vi "Dashboard Main.vi"() -> ()   [LabVIEW 2015]
uses:
  <vilib>/Utility/miscctls.llb/LVRowAndColumnTypeDef.ctl
  <vilib>/event_ctls.llb/eventvkey.ctl
  <vilib>/Rock Robotics/WPI/Dashboard/WPI_DashboardLogging Global.vi
  <vilib>/Rock Robotics/Network Tables/NT Write String Array.vi
  <vilib>/Rock Robotics/Network Tables/NT Read Numeric Array.vi
  <vilib>/Utility/config.llb/Write Key (String).vi
  <vilib>/Utility/config.llb/Write Key (I32).vi
  <vilib>/Rock Robotics/Network Tables/NT Write Boolean.vi
  <vilib>/Rock Robotics/Network Tables/NT Read Boolean.vi
  <vilib>/Utility/config.llb/NI_LVConfig.lvlib
panel:
  in  "TCP":refnum<k5>
  in  "Rec Mode":enum32{"Stop", "Record", "Playback"}(radio)
  in  "Vision":u16(ring) items=["Camera Off", "USB Camera SW", "USB Camera HW", "IP Camera"]
  out "Camera IP":string
  out "Image Message":string="Timeout in Camera Communications"
  in  "Dashboard Tab":T1(tab)
  in  "Select Auto":string(combo)
  out "NT Connection":bool
  in  "Camera Settings":T2={"Frame Rate"=30, "Compression"=30, "Size"=1} {"Frame Rate" scale=1.0..30.0; "Size" items=["640x480", "320x240", "160x120"]}
  out "MotorChart R":cluster{"Numeric":dbl, "Numeric":dbl}(graph)
  out "MotorChart L":T3(graph)
  out "MotorSliders R":cluster{"MotorSlide1":dbl, "MotorSlide2":dbl} {"MotorSlide2" scale=-1.0..1.0 scale format="%#_2e"; "MotorSlide1" scale=-1.0..1.0 scale format="%#_2e"}
  out "MotorSliders L":T4 {"MotorSlide4 2" scale=0.0..14.0 scale format="%#_2e"; "MotorSlide2" scale=-1.0..1.0 scale format="%#_2e"; "MotorSlide1" scale=-1.0..1.0 scale format="%#_2e"}
  out "Gyro":dbl(knob) scale=0.0..360.0
  out "JS1 Z":dbl(slide) scale=-1.0..1.0 scale format="%#_2e"
  out "JS1 Graph":cluster{"X":dbl, "Y":dbl}[](graph)
  out "JS1 Buttons":T5
  out "JS2 Z":dbl(slide) scale=-1.0..1.0 scale format="%#_2e"
  out "JS2 Graph":cluster{"X":dbl, "Y":dbl}[](graph)
  out "JS2 Buttons":T5
  out "Mode":T6(ring)=enum."Auto Disabled"
  in  "DB Camera Config":bool
  out "fps":dbl format="%#.1g"
  out "Mbps":dbl format="%#.1g"
  out "Mbps LED":bool
  in  "File Name":string(combo)
  in  "Key":string[][](array[string])
  in  "Test":bool
  out "Lights Connected":bool
  in  "Test Slider":dbl(slide) scale=0.0..100.0 scale format="%#_3g"
  in  "On/Off":bool caption="Solenoid"
  in  "Test Name":u16(ring) items=["Select the test to run..."]
  in  "Test Tree":string(tree)
  in  "Motor":cluster{"Value":dbl, "Enable":bool} {"Value" scale=-1.0..1.0 scale format="%#_3g"}
  out "Progress":T7 {"Test Progress" scale=0.0..100.0}
  in  "Rev/Fwd":cluster{"Forward":bool, "Reverse":bool}
  in  "Test Ring":u16(ring) items=["Monochrome", "Color"]
  out "Cmd Status":string
  in  "Execute Command":bool
  in  "Command Params":string[][](table)
  in  "Command Selection":i32(listbox)
  in  "CheckList":i32(listbox)
  out "Tree":string(tree)
  out "Camera Image":T8(plugin-control)
  out "Background":bool
  # "Left"
  # "Front"
  # "Right"
  # "Battery"
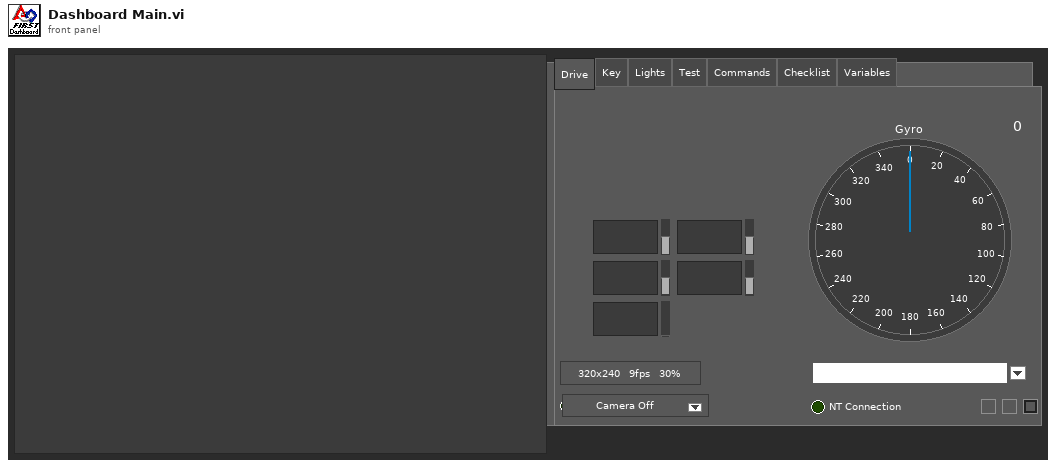
[diagram p1: front panel]
types:
  T1 = enum32{"Drive", "Key", "Lights", "Test", "Commands", "Checklist", "Variables"}
  T2 = cluster{"Frame Rate":i32, "Compression":i32, "Size":u16}
  T3 = cluster{"Numeric":dbl, "Numeric":dbl, "Battery V":dbl}
  T4 = cluster{"MotorSlide1":dbl, "MotorSlide2":dbl, "MotorSlide4 2":dbl}
  T5 = cluster{bool, bool, bool, bool, bool, bool, bool, bool, bool, bool, bool, bool}
  T6 = enum8{"Tele-Op Disabled", "Tele-Op Enabled", "Auto Disabled", "Auto Enabled", "Test Disabled", "Test Enabled", "Disconnected", "No Code", "E-Stop"}
  T7 = cluster{"Test Progress":u8, "Test Progress Text":string}
  T8 = typedef "IMAQ Image.ctl" = refnum<image>
  T9 = cluster{"IDs":cluster{"RPC field ID":u16, "Unique ID":u16}, "String":string}
  T10 = enum32{"Drive", "Basic", "Custom", "Test", "Checklist", "Variables"}
  T11 = typedef "Image Type" = u32
  T12 = cluster{"Camera Image":refnum<vi>, "Dashboard Tab":refnum<vi>, "Background":refnum<vi>, "Vision":refnum<vi>, "Rec Mode":refnum<vi>, "Test Slider":refnum<vi>, "On/Off ":refnum<vi>, "Test Ring":refnum<vi>, "Rev/Fwd":refnum<vi>, "Test Name":refnum<vi>, "Motor":refnum<vi>, "Progress":refnum<vi>, "CheckList":refnum<vi>, "Tree":refnum<vi>, "Test Tree":refnum<vi>, "Command Params":refnum<vi>, "Command Selection":refnum<vi>, "Execute Command":refnum<vi>, "Cmd Status":refnum<vi>}
  T13 = cluster{"Error Strings":string, "Disable Counts":cluster{u16, u16}, "Rail Faults":cluster{u16, u16, u16}, "Robot IP":string, "DB Mode":u8, "Event Info":cluster{"Name":string, "Type":u8, "Number":u16, "Replay":u8}, "Camera Addr":string}
  T14 = cluster{"Storage":cluster{"Disk Free":u64, "RAM Block":u32, "RAM free":u32}, "CPU Utilization":cluster{"CPU % ISR":sgl, "CPU % Time Crit":sgl, "CPU % Timed Str":sgl, "CPU % High":sgl, "CPU % Above":sgl, "CPU % Normal":sgl, "CPU % Low":sgl}, "CAN":cluster{"% Bus Utilization":sgl, "Bus Off Cnt":u32, "TX_FIFO Full Cnt":u32, "Receive Error Cnt":u8, "Transmit Error Cnt":u8}, "HID":cluster{"HID Outputs":u32, "Rumble Low":u16, "Rumble High":u16}[]}
  T15 = cluster{"Status bits":cluster{"Test Mode":bool, "Autonomous":bool, "Enabled":bool, "Code Start":bool, "Brownout":bool, "Reserved 2":bool, "Reserved 3":bool, "E-Stop":bool}, "Code Trace":cluster{"Disabled":bool, "TeleOp":bool, "Auto":bool, "Test":bool}, "Controller Type":enum16{"unknown", "cRIO", "roboRio"}, "Code?":enum16{"unknown", "noCode", "code"}, "Battery V":dbl}
  T16 = cluster{"Control Bits":cluster{"TestMode":bool, "Autonomous":bool, "Enabled":bool, "FMS Present":bool, bool, bool, bool, "E-Stop":bool}, "Team Station ":u8, "Countdown":sgl, "Joystick Values":cluster{"Axes":dbl[], "Buttons":bool[], "POVs":i16[]}[]}
  T17 = cluster{"Axes":dbl[], "Buttons":bool[], "POVs":i16[]}[]
  T18 = cluster{"Axes":dbl[], "Buttons":bool[], "POVs":i16[]}
  T19 = cluster{"Buttons[0]":bool, "Buttons[1]":bool, "Buttons[2]":bool, "Buttons[3]":bool, "Buttons[4]":bool, "Buttons[5]":bool, "Buttons[6]":bool, "Buttons[7]":bool, "Buttons[8]":bool, "Buttons[9]":bool, "Buttons[10]":bool, "Buttons[11]":bool}
  T20 = typedef "NI_LVConfig.lvlib/Config Data RefNum.ctl" = refnum<k1>
  T21 = cluster{"Operation":enum16{"Update", "Clear"}, "Color Box":u32}[]
  T22 = typedef "eventvkey.ctl" = enum16{"ASCII", "Enter", "Return", "Shift", "Ctrl", "Alt", "Cmd", "Opt", "Caps", "NumLock", "Clear", "Break", "Up", "Down", "Left", "Right", "Insert", "Delete", "Home", "End", "PageUp", "PageDown", "Escape", "Help", "Pause", "ScrollLock", "F1", "F2", "F3", "F4", "F5", "F6", "F7", "F8", "F9", "F10", "F11", "F12", "F13", "F14", "F15", "F16", "F17", "F18", "F19", "F20", "F21", "F22", "F23", "F24", "Play", "VolumeUp", "VolumeDown", "Mute", "Two Byte Char"}
  T23 = cluster{"Image Size":bool, "Image Type":bool, "Pixel Value":bool, "ROI Information":bool, "Zoom Factor":bool}
  T24 = enum8{"Enabled", "Disabled", "Disabled and Grayed Out"}
  T25 = cluster{"Operation":enum16{"Update", "Clear"}, "Color Box":u32}
  T26 = typedef "LVRowAndColumnTypeDef.ctl" = cluster{"Row":i32, "Column":i32}
  T27 = cluster{"Shift":bool, "Ctrl":bool, "Alt":bool, "Cmd":bool, "Opt":bool}
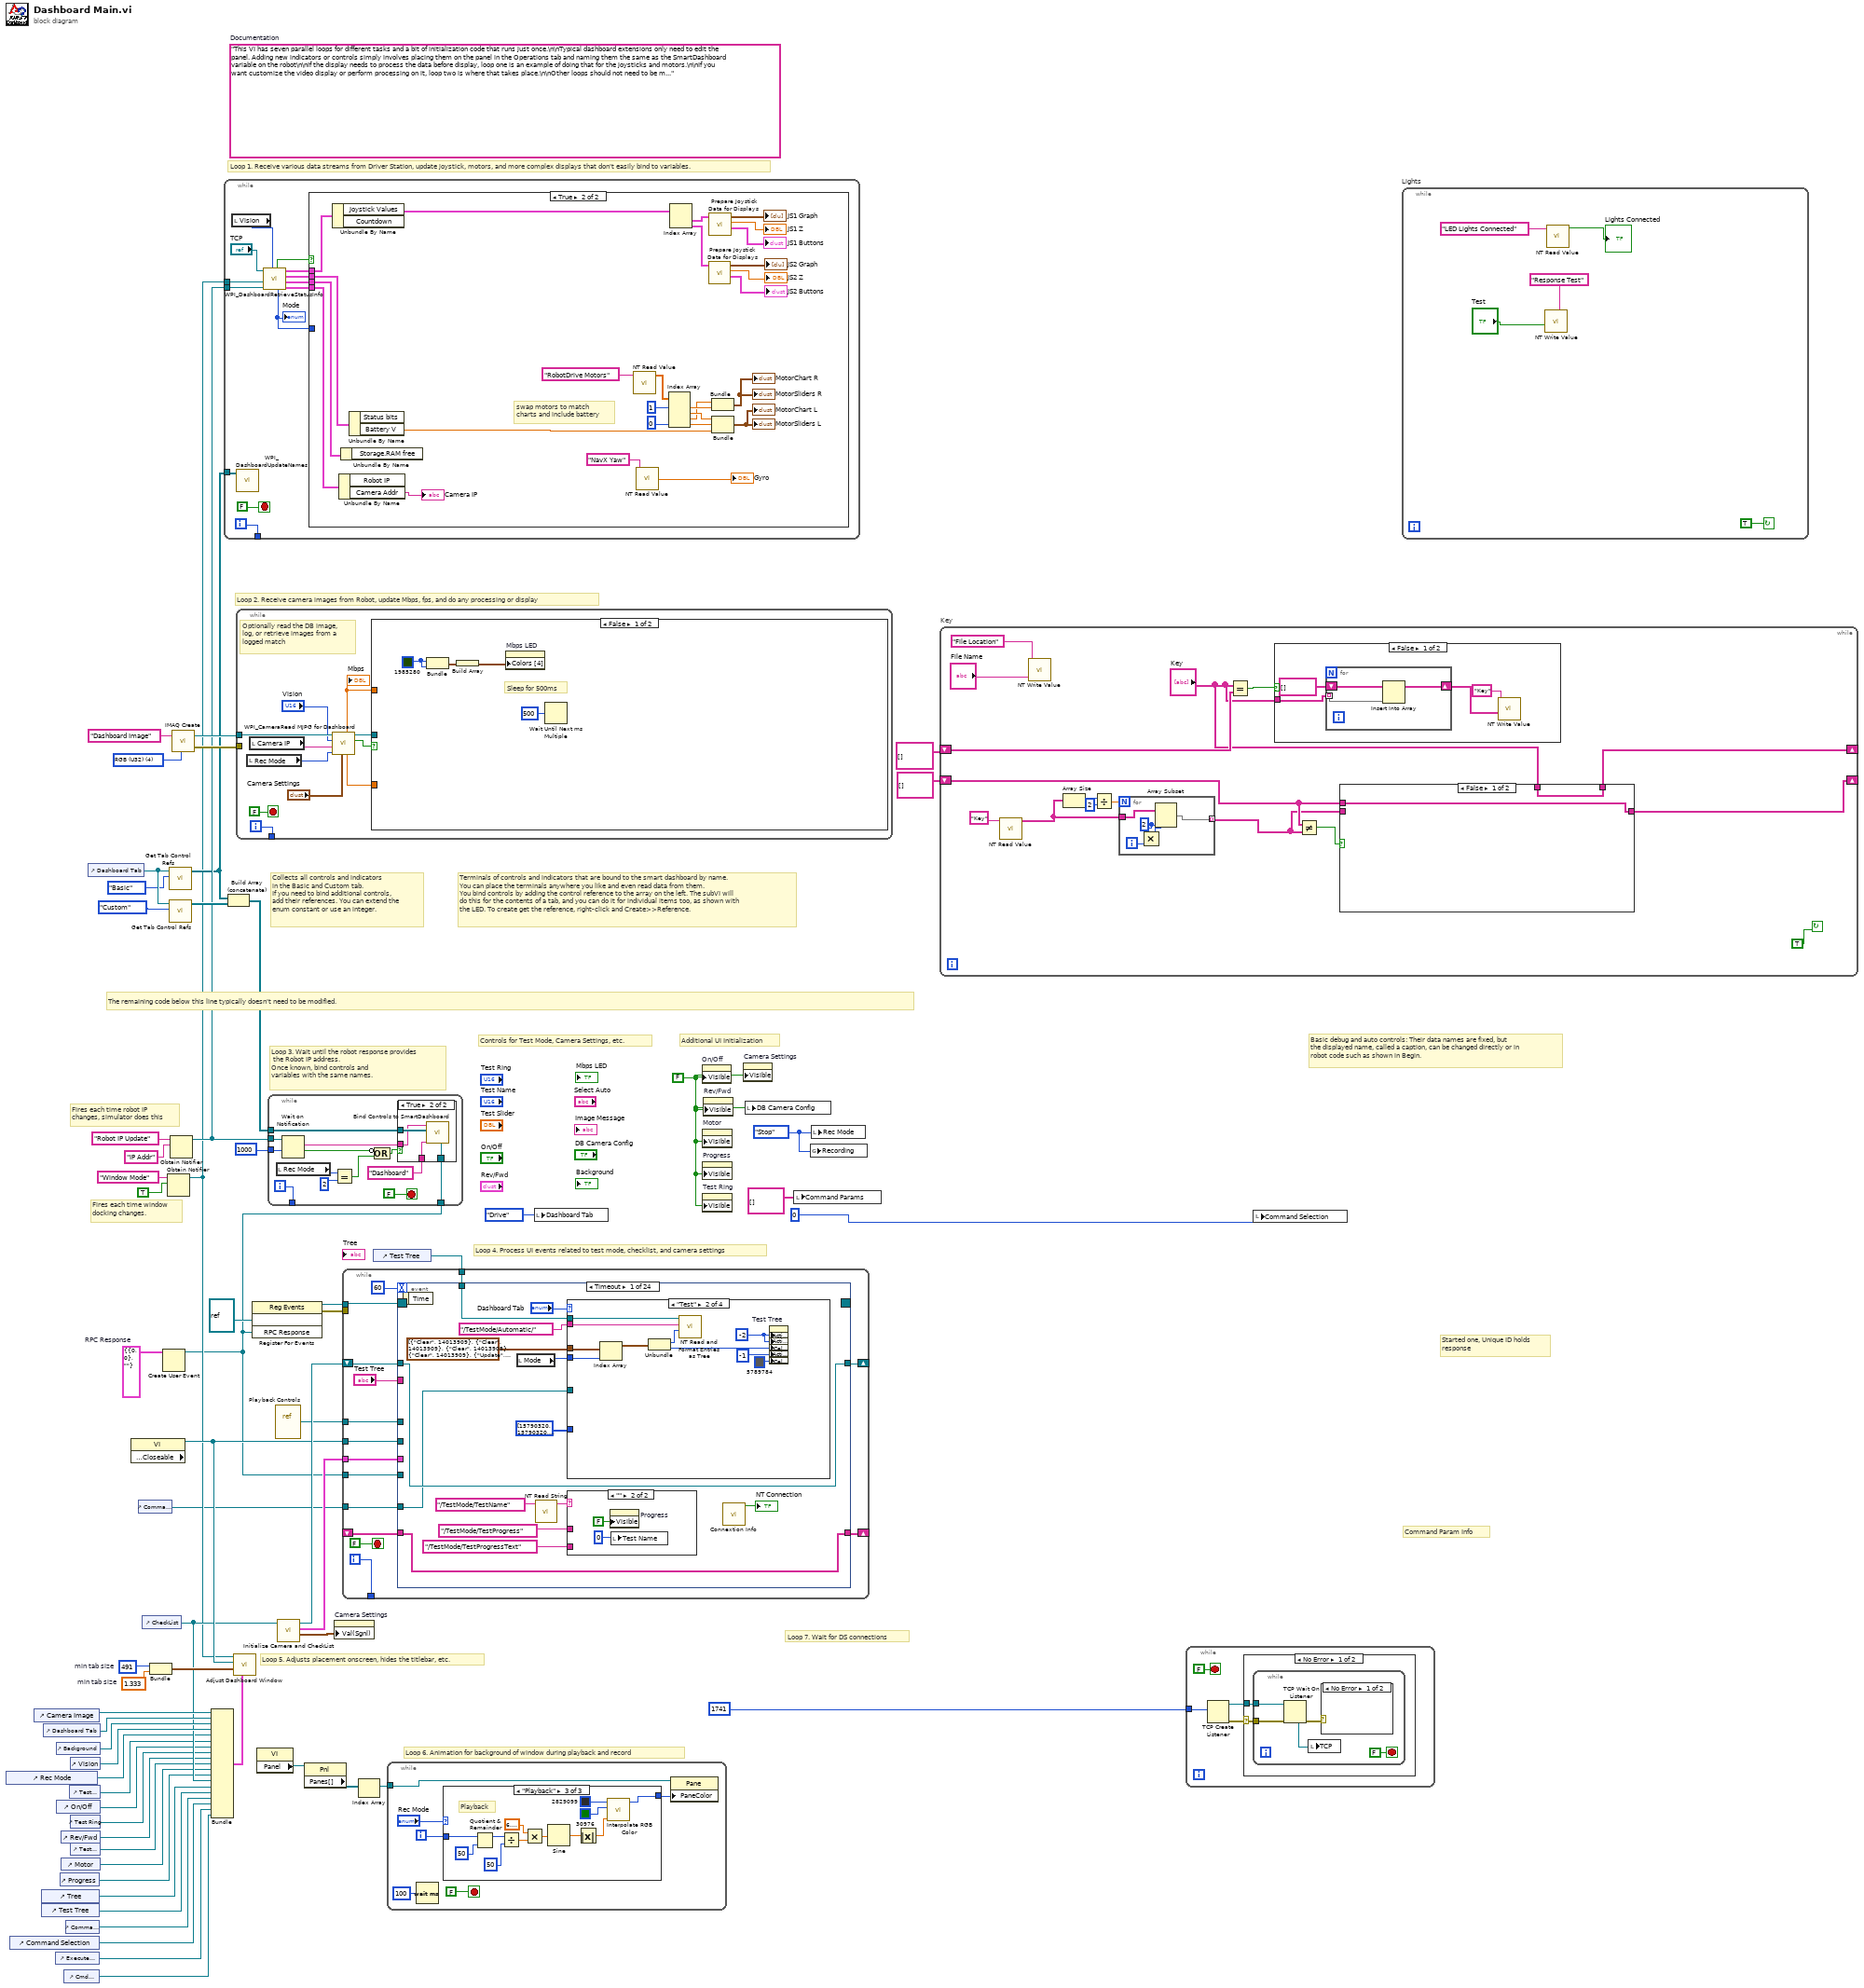
[diagram p0: block diagram]
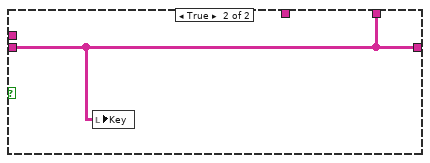
[diagram p2: hidden frame]
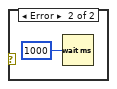
[diagram p4: hidden frame]
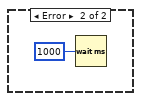
[diagram p5: hidden frame]
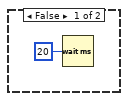
[diagram p6: hidden frame]
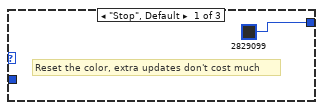
[diagram p7: hidden frame]
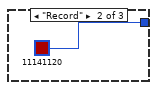
[diagram p8: hidden frame]
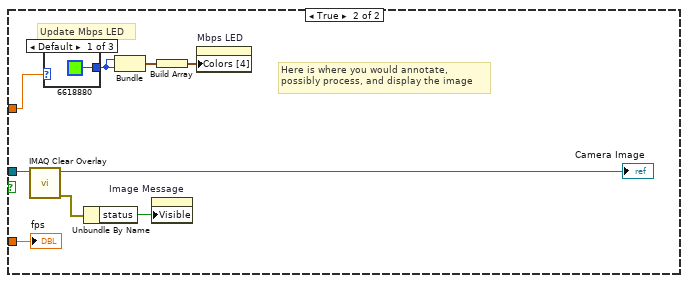
[diagram p10: hidden frame]
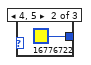
[diagram p11: hidden frame]
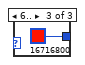
[diagram p12: hidden frame]
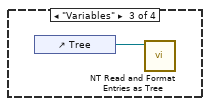
[diagram p14: hidden frame]
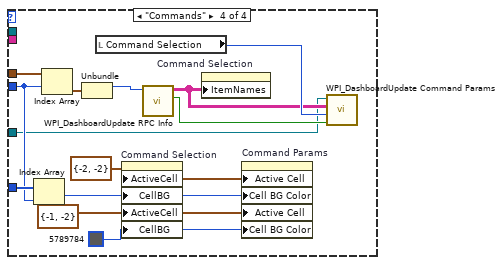
[diagram p15: hidden frame]
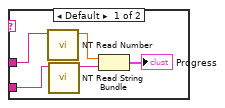
[diagram p16: hidden frame]
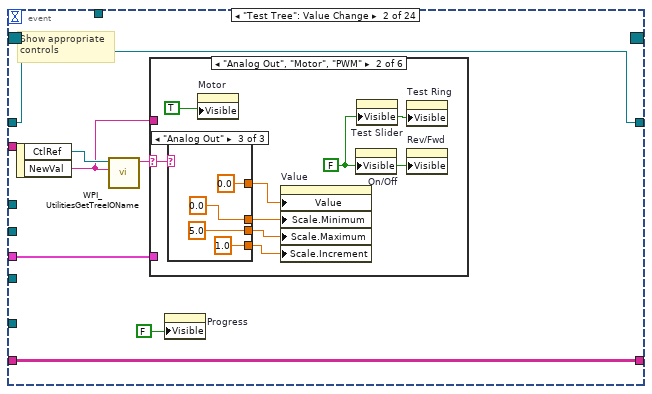
[diagram p17: hidden frame]
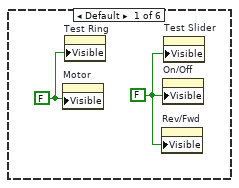
[diagram p18: hidden frame]
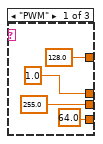
[diagram p19: hidden frame]
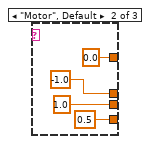
[diagram p20: hidden frame]
diagram:
  w9 = T9 {"IDs"={"RPC field ID"=0, "Unique ID"=0}, "String"=""}  # RPC Response
  w35 = 491  # min tab size
  w34 = 1.333  # min tab size
  w43 = enum32{"Stop", "Record", "Playback"}."Stop" ("Rec Mode")
  w17 = FALSE ("Visible")
  (unwired) "This VI has seven parallel loops for different tasks and a bit of initialization code that runs just once.\n\nTypical dashboard extensions only need to edit the panel. Adding new indicators or controls simply involves placing them on the panel in the Operations tab and naming them the same as the SmartDashboard variable on the robot\n\nIf the display needs to process the data before display, loop one is an example of doing that for the joysticks and motors.\n\nIf you want customize the video display or perform processing on it, loop two is where that takes place.\n\nOther loops should not need to be modified. They are pretty standard, and document the task they perform."  # Documentation
  w63 = T11 4 items=["Grayscale (U8)", "Grayscale (I16)", "Grayscale (SGL)", "Complex (CSG)", "RGB (U32)", "HSL (U32)", "RGB (U64)"] ("Image Type")
  # "Command Param Info"
  # "Started one, Unique ID holds\nresponse"
  # "Loop 7. Wait for DS connections"
  # "Basic debug and auto controls: Their data names are fixed, but\nthe displayed name, called a caption, can be changed directly or in\nrobot code such as shown in Begin."
  # "Controls for Test Mode, Camera Settings, etc."
  # "Additional UI Initialization"
  # "Loop 6. Animation for background of window during playback and record"
  # "Fires each time robot IP\nchanges, simulator does this"
  # "Fires each time window\ndocking changes."
  # "Collects all controls and indicators\nin the Basic and Custom tab.\nIf you need to bind additional controls,\nadd their references. You can extend the\nenum constant or use an integer."
  # "The remaining code below this line typically doesn't need to be modified."
  # "Loop 4. Process UI events related to test mode, checklist, and camera settings"
  # "Terminals of controls and indicators that are bound to the smart dashboard by name.\nYou can place the terminals anywhere you like and even read data from them.\nYou bind controls by adding the control reference to the array on the left. The subVI will\ndo this for the contents of a tab, and you can do it for individual items too, as shown with\nthe LED. To create get the reference, right-click and Create>>Reference."
  # "Loop 3. Wait until the robot response provides\n the Robot IP address.\nOnce known, bind controls and\nvariables with the same names."
  # "Loop 5. Adjusts placement onscreen, hides the titlebar, etc."
  # "Loop 1. Receive various data streams from Driver Station, update joystick, motors, and more complex displays that don't easily bind to variables."
  # "Loop 2. Receive camera images from Robot, update Mbps, fps, and do any processing or display"
  n1 = control-ref of="Rec Mode"() -> (w23:refnum<vi>)
  n2 = control-ref of="Command Selection"() -> (w8:refnum<vi>)
  n3 = control-ref of="Camera Image"() -> (w38:refnum<vi>)
  n4 = control-ref of="Tree"() -> (w27:refnum<vi>)
  n5 = control-ref of="Test Tree"() -> (w26:refnum<vi>)
  n6 = control-ref of="Dashboard Tab"() -> (w37:refnum<vi>)
  n7 = control-ref of="Execute Command"() -> (w10:refnum<vi>)
  n8 = control-ref of="Background"() -> (w32:refnum<vi>)
  n9 = control-ref of="On/Off"() -> (w21:refnum<vi>)
  n10 = control-ref of="Progress"() -> (w18:refnum<vi>)
  n11 = control-ref of="Rev/Fwd"() -> (w19:refnum<vi>)
  n12 = control-ref of="Motor"() -> (w24:refnum<vi>)
  n13 = control-ref of="Cmd Status"() -> (w4:refnum<vi>)
  n14 = control-ref of="Command Params"() -> (w11:refnum<vi>)
  n15 = control-ref of="Test Slider"() -> (w22:refnum<vi>)
  n16 = control-ref of="Vision"() -> (w36:refnum<vi>)
  n17 = control-ref of="Test Ring"() -> (w20:refnum<vi>)
  n18 = control-ref of="Test Name"() -> (w25:refnum<vi>)
  n19 = control-ref of="Dashboard Tab"() -> (w41:refnum<vi>)
  n20 = property class="VI" props=["Front Panel.Closeable"]() -> (reference out=w42:refnum<vi>)  [unwired: 2 in, 2 out]
  n21 = control-ref of="Command Params"() -> (w3:refnum<vi>)
  n22 = control-ref of="CheckList"() -> (w28:refnum<vi>)
  n23 = Bundle("min tab size"=w35, "min tab size"=w34) -> (w33:cluster{"min tab size":i32, "min tab size":dbl})  [unwired: 1 in]
  n24 = Create User Event(user event datatype=w9) -> (user event=w5:refnum<user-event>)  [unwired: 1 in, 1 out]
  n25 = Obtain Notifier(name (unnamed)="Window Mode", notification data type=TRUE) -> (notifier out=w14:refnum<notifier>)  [unwired: 2 in, 2 out]
  n26 = call <vilib>:"Get Tab Control Refs.vi"("Page Index"=T10."Basic" ("Dashboard Tab"), "TabControl in"=w41) -> ("ControlsOnPage"=w15:refnum<vi>[])  [unwired: 9 in]
  n27 = call <vilib>:"Get Tab Control Refs.vi"("Page Index"=T10."Custom" ("Dashboard Tab"), "TabControl in"=w41) -> ("ControlsOnPage"=w40:refnum<vi>[])  [unwired: 9 in]
  n28 = Obtain Notifier(name (unnamed)="Robot IP Update", notification data type="IP Addr" ("name (unnamed)")) -> (notifier out=w16:refnum<notifier>)  [unwired: 2 in, 2 out]
  n29 = call "IMAQ Create"("Image Name"="Dashboard Image", "Image Type"=w63) -> ("New Image"=w61:T8, "error out"=w60:errorcluster)  [unwired: 2 in, 1 out]
  n30 = Bundle("Camera Image"=w38, "Dashboard Tab"=w37, "Background"=w32, "Vision"=w36, "Rec Mode"=w23, "Test Slider"=w22, "On/Off"=w21, "Test Ring"=w20, "Rev/Fwd"=w19, "Test Name"=w25, "Motor"=w24, "Progress"=w18, "CheckList"=w28, "Tree"=w27, "Test Tree"=w26, "Command Params"=w11, "Command Selection"=w8, "Execute Command"=w10, "Cmd Status"=w4) -> (w29:T12)  [unwired: 1 in]
  n31 = while {
    tunnel: [w75] -> _
    tunnel: w16 -> [w69]
    tunnel: w15 -> [w68]
    tunnel: w14 -> [w64]
    i -> [w75]
    stop <- FALSE stop-if-true
    n32 = local read "Vision"() -> (w66:u16)
    n33 = call <vilib>:"WPI_DashboardUpdateNames.vi"("Controls on Tab"=w68) -> ()  [unwired: 11 in]
    n34 = call <vilib>:"WPI_DashboardRetrieveStatusInfo.vi"("Vision"=w66, "Binding Refnum"=w69, "Window Mode Notifier"=w64, "TCP Cnx"="TCP") -> ("Power and Errors"=w70:T13, "Robot Metrics"=w73:T14, "Status Info"=w74:T15, "Control Info"=w71:T16, "Robot Mode"=w67:T6, "Process?"=w72:bool)  [unwired: 2 in]
    "Mode" <- w67
    n35 = case shown="True" w72 {
      tunnel: w74 -> [_ w104]
      tunnel: w73 -> [_ w103]
      tunnel: w71 -> [_ w102]
      tunnel: w70 -> [_ w101]
      tunnel: w67 -> [_ _]
      frame False {
        n36 = Wait (ms)(milliseconds to wait=u32 20) -> ()  [unwired: 1 out]
      }
      frame True {
        # "swap motors to match\ncharts and include battery"
        n37 = Unbundle By Name(w102) -> ("Joystick Values"=w91:T17)  [unwired: 1 out]
        n38 = Unbundle By Name(w101) -> ("Camera Addr"=→"Camera IP":string)  [unwired: 1 out]
        n39 = Unbundle By Name(w103) -> ()  [unwired: 1 out]
        n40 = Unbundle By Name(w104) -> ("Battery V"=w92:dbl)  [unwired: 1 out]
        n41 = call-poly <vilib>:"NT Read Value.vi"("Name"="RobotDrive Motors") -> ("Numeric Array"=w80:dbl[])  [unwired: 9 in, 1 out]
        n42 = call-poly <vilib>:"NT Read Value.vi"("Name"="NavX Yaw") -> ("Numeric"=→"Gyro":dbl)  [unwired: 9 in, 1 out]
        n43 = Index Array(array=w80, index #1=1, index #4=0) -> (element #1=w96:dbl, element #2=w97:dbl, element #3=w95:dbl, element #4=w100:dbl)  [unwired: 2 in]
        n44 = Index Array(array=w91) -> (element #1=w90:T18, element #2=w85:T18)  [unwired: 2 in]
        n45 = call "Prepare Joystick Data for Displays.vi"("Joystick Values"=w85) -> ("Buttons"=→"JS2 Buttons":T19, "Z Axis"=→"JS2 Z":dbl, "Cartesian Data"=→"JS2 Graph":cluster{"X axis":dbl, "X axis":dbl}[])  [unwired: 8 in]
        n46 = call "Prepare Joystick Data for Displays.vi"("Joystick Values"=w90) -> ("Buttons"=→"JS1 Buttons":T19, "Z Axis"=→"JS1 Z":dbl, "Cartesian Data"=→"JS1 Graph":cluster{"X axis":dbl, "X axis":dbl}[])  [unwired: 8 in]
        n47 = Bundle("Numeric"=w95, "Numeric"=w96) -> (→"MotorChart R" →"MotorSliders R":cluster{"Numeric":dbl, "Numeric":dbl})  [unwired: 1 in]
        n48 = Bundle("Numeric"=w97, "Numeric"=w100, "Battery V"=w92) -> (→"MotorChart L" →"MotorSliders L":T3)  [unwired: 1 in]
      }
    }
  }
  n49 = Build Array (concatenate)(w15, w40) -> (w39:refnum<vi>[])
  n50 = call "Adjust Dashboard Window.vi"("Sizing Refnums"=w29, "Size Constraints"=w33, "VI"=w42, "WIn Mode"=w14) -> ()  [unwired: 8 in]
  n51 = while {
    tunnel: w61 -> [w113]
    tunnel: w60 -> [_]
    tunnel: [w114] -> _
    i -> [w114]
    stop <- FALSE stop-if-true
    # "Optionally read the DB image,\nlog, or retrieve images from a\nlogged match"
    n52 = local read "Rec Mode"() -> (w108:enum32{"Stop", "Record", "Playback"})
    n53 = local read "Camera IP"() -> (w106:string)
    n54 = call <vilib>:"WPI_CameraRead MJPG for Dashboard.vi"("Camera Settings"="Camera Settings", "Rec Mode"=w108, "Camera IP"=w106, "Camera Mode"="Vision", "Refnum in"=w113) -> ("Active"=w111:bool, "Refnum out"=w112:T8, "FPS"=w110:dbl, "Bandwidth (Mbps)"=w105:dbl)  [unwired: 3 in]
    "Mbps" <- w105
    n55 = case shown="False" w111 {
      tunnel: w112 -> [_ w123]
      tunnel: w105 -> [_ w122]
      tunnel: w110 -> [_ w120]
      frame False {
        w116 = u32 1985280 ("Color Box")
        # "Sleep for 500ms"
        n56 = Bundle("Color Box"=w116, "Color Box"=w116) -> (w118:cluster{"Color Box":u32, "Color Box":u32})  [unwired: 1 out]
        n57 = Build Array(w118) -> (w117:cluster{"Color Box":u32, "Color Box":u32}[])
        n58 = property on="Mbps LED" class="Bool (strict)"("Colors [4]"=w117) -> ()  [unwired: 2 in, 2 out]
        n59 = Wait Until Next ms Multiple(millisecond multiple=u32 500) -> ()  [unwired: 1 out]
      }
      frame True {
        # "Here is where you would annotate,\npossibly process, and display the image"
        # "Update Mbps LED"
        n60 = call "IMAQ Clear Overlay"("Image"=w123) -> ("error out"=w127:errorcluster, "Image Out"=→"Camera Image":T8)  [unwired: 2 in, 7 out]
        n61 = case shown="Default" w122 {
          tunnel: [u32 6618880 ("Color Box") u32 16776722 ("Color Box") u32 16716800 ("Color Box")] -> w124
          frame Default {
          }
          frame 4, 5 {
          }
          frame 6.. {
          }
        }
        n62 = Unbundle By Name(w127) -> ("status"=w128:bool)
        n63 = Bundle("Color Box"=w124, "Color Box"=w124) -> (w126:cluster{"Color Box":u32, "Color Box":u32})  [unwired: 1 out]
        n64 = property on="Image Message" class="Str"("Visible"=w128) -> ()  [unwired: 2 in, 2 out]
        n65 = Build Array(w126) -> (w125:cluster{"Color Box":u32, "Color Box":u32}[])
        n66 = property on="Mbps LED" class="Bool (strict)"("Colors [4]"=w125) -> ()  [unwired: 2 in, 2 out]
        "fps" <- w120
      }
    }
  }
  n67 = register-events(refnum<vi> refnum, w5) -> (reference out=w47:refnum<event-registration>, error out=w46:errorcluster)  [unwired: 2 in]
  n68 = property class="VI"() -> ("Panel"=w50:refnum<vi>)  [unwired: 2 in, 2 out]
  n69 = while {
    tunnel: w39 -> [w144]
    tunnel: w16 -> [w142]
    tunnel: [w140] -> _
    tunnel: u32 1000 ("milliseconds to wait") -> [w139]
    tunnel: w5 -> [w132]
    i -> [w140]
    stop <- FALSE stop-if-true
    n70 = local read "Rec Mode"() -> (w135:enum32{"Stop", "Record", "Playback"})
    n71 = Wait on Notification(notifier=w142, timeout in ms (-1)=w139) -> (notification=w141:string, timed out?=w137:bool)  [unwired: 2 in, 2 out]
    n72 = Equal?(x=w135, y=u16 2 ("Rec Mode")) -> (x = y?=w136:bool)
    n73 = Compound Arithmetic op=OR(invert w137, w136) -> (w138:bool)
    n74 = case shown="True" w138 {
      tunnel: w144 -> [_ w148]
      tunnel: w141 -> [_ w147]
      tunnel: "Dashboard" -> [_ w146]
      tunnel: w132 -> [_ w145]
      frame False {
      }
      frame True {
        n75 = call <vilib>:"Bind Controls to SmartDashboard.vi"("RPC ref"=w145, "Client Name"=w146, "Bound Control Refs"=w148, "Server IP Address"=w147) -> ()  [unwired: 8 in]
      }
    }
  }
  n76 = vi-ref "Playback Controls.vi"() -> (w48:refnum<vi>)
  n77 = call "Initialize Camera and CheckList.vi"("ListBox in"=w28) -> ("Cluster"=w54:cluster{"value":i32, "value":i32, "index":i32}, "Array"=w55:cluster{string[]}[], "File Refnum"=w53:T20)  [unwired: 8 in]
  n78 = property class="Pnl"(reference=w50) -> ("Panes[]"=w51:refnum<vi>[])  [unwired: 1 in, 2 out]
  n79 = property on="Camera Settings" class="Clust (strict)"("Val(Sgnl)"=w54) -> ()  [unwired: 2 in, 2 out]
  n80 = Index Array(array=w51) -> (element=w49:refnum<vi>)  [unwired: 1 in]
  n81 = control-ref of="Test Tree"() -> (w52:refnum<vi>)
  n82 = while {
    tunnel: w55 -> [w160]
    shift-right: [w159] -> _
    shift-left: w53 -> [w158]
    tunnel: [w157] -> _
    tunnel: w52 -> [w156]
    tunnel: w48 -> [w155]
    tunnel: w47 -> [w154]
    tunnel: w46 -> [_]
    tunnel: w42 -> [w153]
    tunnel: w5 -> [w152]
    tunnel: w3 -> [w151]
    shift-right: [w150] -> _
    shift-left: _ -> [w149]
    i -> [w157]
    stop <- FALSE stop-if-true
    n83 = event shown="[0] Timeout" {
      selector: w154 -> [_ _ _ _ _ _ _ _ _ _ _ _ _ _ _ _ _ _ _ _ _ _ _ _]
      dyn-events: [_ _ _ _ _ _ _ _ _ _ _ _ _ _ _ _ _ _ w469 _ _ _ _ _] -> _
      timeout: u32 60 ("milliseconds to wait") -> [_ _ _ _ _ _ _ _ _ _ _ _ _ _ _ _ _ _ _ _ _ _ _ _]
      tunnel: w156 -> [w173 _ _ _ _ _ _ _ _ _ _ _ _ _ _ _ _ _ _ _ _ _ _ _]
      tunnel: "Test Tree" -> [_ _ _ _ _ _ _ _ _ _ _ _ _ w432 w441 w444 w449 w458 _ _ _ _ _ _]
      tunnel: w160 -> [_ w211 _ _ _ _ _ _ _ _ _ w394 w425 _ _ _ _ _ _ _ _ _ _ _]
      tunnel: [w170 w210 w314 w320 w330 w334 w340 w352 w360 w366 w379 w393 w418 w431 w439 w443 w448 w457 w471 w487 w489 w497 w508 w513] -> w159
      tunnel: w158 -> [w170 w210 w314 w320 w330 w334 w340 w352 w360 w366 w379 w392 w418 w431 w439 w443 w448 w457 w471 w487 w489 w497 w508 w513]
      tunnel: w155 -> [_ _ _ _ _ _ _ _ _ _ _ _ _ _ _ _ _ _ w472 _ w492 _ _ _]
      tunnel: w153 -> [_ _ _ _ _ _ _ _ _ _ _ _ _ _ _ _ _ _ w467 _ _ _ _ _]
      tunnel: w152 -> [_ _ _ _ _ _ _ _ _ _ _ _ _ _ _ _ _ _ w463 _ _ _ _ _]
      tunnel: w151 -> [w165 _ _ _ _ _ w338 _ _ _ _ _ _ _ _ _ _ _ _ _ _ _ _ _]
      tunnel: [w164 w209 w313 w319 w329 w335 w336 w346 w357 w365 w378 w391 w417 w430 w438 w442 w447 w456 w462 w485 w488 w493 w501 w514] -> w150
      tunnel: w149 -> [w164 w209 w313 w319 w329 w335 w336 _ _ w365 w378 w391 w417 w430 w438 w442 w447 w456 w462 w485 w488 w493 w501 w514]
      event Timeout {
        n84 = event-data() -> ()  [unwired: 1 in, 1 out]
        n85 = local read "Mode"() -> (w167:T6)
        n86 = call <vilib>:"NT Read String.vi"("Name"="/TestMode/TestName") -> ("String"=w176:string)  [unwired: 9 in, 1 out]
        n87 = case shown="\"Test\"" "Dashboard Tab" {
          tunnel: w173 -> [_ w187 _ _]
          tunnel: "/TestMode/Automatic/" ("Name Pattern") -> [_ w186 _ _]
          tunnel: T21 [{"Operation"=enum."Clear", "Color Box"=14013909}, {"Operation"=enum."Clear", "Color Box"=14013909}, {"Operation"=enum."Clear", "Color Box"=14013909}, {"Operation"=enum."Clear", "Color Box"=14013909}, {"Operation"=enum."Update", "Color Box"=14013909}, {"Operation"=enum."Update", "Color Box"=16777215}, {"Operation"=enum."Clear", "Color Box"=14013909}, {"Operation"=enum."Clear", "Color Box"=14013909}, {"Operation"=enum."Clear", "Color Box"=14013909}] -> [_ w179 _ w196]
          tunnel: w167 -> [_ w178 _ w195]
          tunnel: u32[] [15790320, 15790320, 15790320, 15790320, 16777215, 16777215, 15790320, 15790320, 15790320] -> [_ _ _ w201]
          tunnel: w165 -> [_ _ _ w189]
          frame "Lights", Default {
          }
          frame "Test" {
            w185 = -2 ("Active Item:Row Number")
            n88 = Index Array(array=w179, index=w178) -> (element=w180:T25)
            n89 = Unbundle(w180) -> ("Operation"=w181:enum16{"Update", "Clear"}, "Color Box"=w182:u32)
            n90 = call <vilib>:"NT Read and Format Entries as Tree.vi"("Operation"=w181, "Name Pattern"=w186, "Tree Refnum"=w187) -> ()  [unwired: 7 in, 2 out]
            n91 = property on="Test Tree" class="Tree (strict)"("Active Item Row Number"=w185, "ActiveColNum"=w185, "CellBG"=w182, "Active Item Row Number"=-1 ("Active Item:Row Number"), "CellBG"=u32 5789784 ("Color Box")) -> ()  [unwired: 2 in, 2 out]
          }
          frame "Variables" {
            n92 = control-ref of="Tree"() -> (w188:refnum<vi>)
            n93 = call <vilib>:"NT Read and Format Entries as Tree.vi"("Tree Refnum"=w188) -> ()  [unwired: 9 in, 2 out]
          }
          frame "Commands" {
            w197 = u32 5789784 ("Color Box")
            w198 = T26 {"Row"=-1, "Column"=-2} ("Active Cell:Active Cell")
            w200 = T26 {"Row"=-2, "Column"=-2} ("Active Cell:Active Cell")
            n94 = Index Array(array=w201, index=w195) -> (element=w199:u32)
            n95 = Index Array(array=w196, index=w195) -> (element=w194:T25)
            n96 = Unbundle(w194) -> ("Operation"=w193:enum16{"Update", "Clear"})  [unwired: 1 out]
            n97 = local read "Command Selection"() -> (w192:i32)
            n98 = property on="Command Selection" class="MCListbox (strict)"("ActiveCell"=w200, "CellBG"=w199, "ActiveCell"=w198, "CellBG"=w197) -> ()  [unwired: 2 in, 2 out]
            n99 = call <vilib>:"WPI_DashboardUpdate RPC Info.vi"("Operation"=w193) -> ("update"=w191:bool, "commands"=w190:string[][])  [unwired: 9 in]
            n100 = property on="Command Selection" class="MCListbox (strict)"("ItemNames"=w190) -> ()  [unwired: 2 in, 2 out]
            n101 = property on="Command Params" class="Tbl (strict)"("Active Cell"=w200, "Cell BG Color"=w199, "Active Cell"=w198, "Cell BG Color"=w197) -> ()  [unwired: 2 in, 2 out]
            n102 = call <vilib>:"WPI_DashboardUpdate Command Params.vi"("Update"=w191, "NewVal"=w192, "Commands"=w190, "Param Tbl"=w189) -> ()  [unwired: 7 in, 1 out]
          }
        }
        n103 = case shown="\"\"" w176 {
          tunnel: "/TestMode/TestProgress" ("Name") -> [w203 _]
          tunnel: "/TestMode/TestProgressText" ("Name") -> [w202 _]
          frame Default {
            n104 = call <vilib>:"NT Read Number.vi"("Name"=w203) -> ("Numeric"=w204:dbl)  [unwired: 9 in, 1 out]
            n105 = call <vilib>:"NT Read String.vi"("Name"=w202) -> ("String"=w205:string)  [unwired: 9 in, 1 out]
            n106 = Bundle("Numeric"=w204, "String"=w205) -> (→"Progress":cluster{"Numeric":dbl, "String":string})  [unwired: 1 in]
          }
          frame "" {
            n107 = property on="Progress" class="Clust (strict)"("Visible"=FALSE) -> ()  [unwired: 2 in, 2 out]
            n108 = local write "Test Name"(u16 0) -> ()
          }
        }
        n109 = call <vilib>:"Connextion Info.vi"() -> ("Connected"=→"NT Connection":bool)  [unwired: 10 in, 1 out]
      }
      event "Test Tree": Value Change {
        # "Show appropriate\ncontrols"
        n110 = event-data() -> ("CtlRef"=w214:refnum<vi>, "NewVal"=w212:string)  [unwired: 1 in]
        n111 = call <vilib>:"WPI_UtilitiesGetTreeIOName.vi"("NewVal"=w212, "TreeControl in"=w214) -> ("I/O Name"=w215:string)  [unwired: 9 in]
        n112 = case shown="\"Analog Out\", \"Motor\", \"PWM\"" w215 {
          selector: w215 -> [_ w222 _ w244 w253 _]
          tunnel: w212 -> [_ _ w241 w243 _ w260]
          tunnel: w211 -> [_ _ _ _ _ w259]
          frame Default {
            w217 = FALSE ("Visible")
            w216 = FALSE ("Visible")
            n113 = property on="Motor" class="Clust (strict)"("Visible"=w216) -> ()  [unwired: 2 in, 2 out]
            n114 = property on="Test Ring" class="Ring (strict)"("Visible"=w216) -> ()  [unwired: 2 in, 2 out]
            n115 = property on="Rev/Fwd" class="Clust (strict)"("Visible"=w217) -> ()  [unwired: 2 in, 2 out]
            n116 = property on="On/Off" class="Bool (strict)"("Visible"=w217) -> ()  [unwired: 2 in, 2 out]
            n117 = property on="Test Slider" class="Slide (strict)"("Visible"=w217) -> ()  [unwired: 2 in, 2 out]
          }
          frame "Analog Out", "Motor", "PWM" {
            w223 = FALSE ("Visible")
            n118 = case shown="\"Analog Out\"" w222 {
              tunnel: [1.0 ("Value") -1.0 ("Value") 0.0 ("Value")] -> w221
              tunnel: [255.0 ("Value") 1.0 ("Value") 5.0 ("Value")] -> w220
              tunnel: [128.0 ("Value") 0.0 ("Value") 0.0 ("Value")] -> w219
              tunnel: [64.0 ("Value") 0.5 ("Value") 1.0 ("Value")] -> w218
              frame "PWM" {
              }
              frame "Motor", Default {
              }
              frame "Analog Out" {
              }
            }
            n119 = property on="Motor" class="Clust (strict)"("Visible"=TRUE) -> ()  [unwired: 2 in, 2 out]
            n120 = property on="Value" class="Slide (strict)"("Value"=w219, "Scale.Minimum"=w221, "Scale.Maximum"=w220, "Scale.Increment"=w218) -> ()  [unwired: 2 in, 2 out]
            n121 = property on="On/Off" class="Bool (strict)"("Visible"=w223) -> ()  [unwired: 2 in, 2 out]
            n122 = property on="Test Slider" class="Slide (strict)"("Visible"=w223) -> ()  [unwired: 2 in, 2 out]
            n123 = property on="Test Ring" class="Ring (strict)"("Visible"=w223) -> ()  [unwired: 2 in, 2 out]
            n124 = property on="Rev/Fwd" class="Clust (strict)"("Visible"=w223) -> ()  [unwired: 2 in, 2 out]
          }
          frame "Servo" {
            w239 = FALSE ("Visible")
            n125 = call <vilib>:"NT Read Number.vi"("Name"=w241) -> ("Numeric"=w240:dbl)  [unwired: 9 in, 1 out]
            n126 = property on="Test Slider" class="Slide (strict)"("Visible"=TRUE, "Scale.Maximum"=170.0 ("Scale.Range:Maximum")) -> ()  [unwired: 2 in, 2 out]
            n127 = local write "Test Slider"(w240) -> ()
            n128 = property on="Motor" class="Clust (strict)"("Visible"=w239) -> ()  [unwired: 2 in, 2 out]
            n129 = property on="Rev/Fwd" class="Clust (strict)"("Visible"=w239) -> ()  [unwired: 2 in, 2 out]
            n130 = property on="On/Off" class="Bool (strict)"("Visible"=w239) -> ()  [unwired: 2 in, 2 out]
            n131 = property on="Test Ring" class="Ring (strict)"("Visible"=w239) -> ()  [unwired: 2 in, 2 out]
          }
          frame "Relay", "Solenoid" {
            w242 = FALSE ("Visible")
            n132 = property on="Motor" class="Clust (strict)"("Visible"=w242) -> ()  [unwired: 2 in, 2 out]
            n133 = property on="Test Slider" class="Slide (strict)"("Visible"=w242) -> ()  [unwired: 2 in, 2 out]
            n134 = Search and Replace String(input string=w243, search string="/Value  **", replace string="/Direction") -> (result string=w249:string)  [unwired: 5 in, 3 out]
            n135 = property on="Test Ring" class="Ring (strict)"("Visible"=w242) -> ()  [unwired: 2 in, 2 out]
            n136 = call <vilib>:"NT Read String.vi"("Name"=w249) -> ("String"=w247:string)  [unwired: 9 in, 1 out]
            n137 = Equal?(x="Both directions", y=w247) -> (x = y?=w245:bool)
            n138 = Not(x=w245) -> (.not. x?=w246:bool)
            n139 = property on="Rev/Fwd" class="Clust (strict)"("Visible"=w245) -> ()  [unwired: 2 in, 2 out]
            n140 = property on="On/Off" class="Bool (strict)"("Visible"=w246, "Caption.Text"=w244) -> ()  [unwired: 2 in, 2 out]
          }
          frame "Compressor", "Digital Out" {
            w252 = FALSE ("Visible")
            # "Get direction and finish"
            n141 = property on="Motor" class="Clust (strict)"("Visible"=w252) -> ()  [unwired: 2 in, 2 out]
            n142 = property on="Test Slider" class="Slide (strict)"("Visible"=w252) -> ()  [unwired: 2 in, 2 out]
            n143 = property on="Test Ring" class="Ring (strict)"("Visible"=w252) -> ()  [unwired: 2 in, 2 out]
            n144 = property on="On/Off" class="Bool (strict)"("Visible"=TRUE, "Caption.Text"=w253) -> ()  [unwired: 2 in, 2 out]
            n145 = property on="Rev/Fwd" class="Clust (strict)"("Visible"=FALSE) -> ()  [unwired: 2 in, 2 out]
          }
          frame "Camera" {
            n146 = call <vilib>:"Get Last Path Segment.vi"("String in"=w260) -> ("String out"=w261:string)  [unwired: 10 in]
            n147 = property on="On/Off" class="Bool (strict)"("Visible"=FALSE) -> ()  [unwired: 2 in, 2 out]
            n148 = property on="Motor" class="Clust (strict)"("Visible"=FALSE) -> ()  [unwired: 2 in, 2 out]
            n149 = property on="Rev/Fwd" class="Clust (strict)"("Visible"=FALSE) -> ()  [unwired: 2 in, 2 out]
            n150 = case shown="\"White Balance  **\"" w261 {
              tunnel: w260 -> [w267 w276 w285 w294 w303 _ w309]
              tunnel: w259 -> [w265 w273 w282 w291 w300 _ _]
              frame "Size  **" {
                n151 = Index Array(array=w265) -> (element=w264:cluster{string[]})  [unwired: 1 in]
                n152 = call <vilib>:"NT Read String.vi"("Name"=w267) -> ("String"=w266:string)  [unwired: 9 in, 1 out]
                n153 = Unbundle(w264) -> (w262:string[])
                n154 = Match First String(2:w262, 3:w266) -> (0:w263:i32)  [unwired: 1 out]
                n155 = property on="Test Ring" class="Ring (strict)"("Value"=w263, "Strings []"=w262) -> ()  [unwired: 2 in, 2 out]
                n156 = property on="Test Ring" class="Ring (strict)"("Visible"=TRUE) -> ()  [unwired: 2 in, 2 out]
                n157 = property on="Test Slider" class="Slide (strict)"("Visible"=FALSE) -> ()  [unwired: 2 in, 2 out]
              }
              frame "White Balance  **" {
                n158 = Index Array(array=w273, index=1) -> (element=w274:cluster{string[]})
                n159 = call <vilib>:"NT Read String.vi"("Name"=w276) -> ("String"=w275:string)  [unwired: 9 in, 1 out]
                n160 = Unbundle(w274) -> (w271:string[])
                n161 = Match First String(2:w271, 3:w275) -> (0:w270:i32)  [unwired: 1 out]
                n162 = property on="Test Ring" class="Ring (strict)"("Value"=w270, "Strings []"=w271) -> ()  [unwired: 2 in, 2 out]
                n163 = property on="Test Ring" class="Ring (strict)"("Visible"=TRUE) -> ()  [unwired: 2 in, 2 out]
                n164 = property on="Test Slider" class="Slide (strict)"("Visible"=FALSE) -> ()  [unwired: 2 in, 2 out]
              }
              frame "Exposure  **" {
                n165 = Index Array(array=w282, index=2) -> (element=w283:cluster{string[]})
                n166 = call <vilib>:"NT Read String.vi"("Name"=w285) -> ("String"=w284:string)  [unwired: 9 in, 1 out]
                n167 = Unbundle(w283) -> (w279:string[])
                n168 = Match First String(2:w279, 3:w284) -> (0:w280:i32)  [unwired: 1 out]
                n169 = property on="Test Ring" class="Ring (strict)"("Value"=w280, "Strings []"=w279) -> ()  [unwired: 2 in, 2 out]
                n170 = property on="Test Ring" class="Ring (strict)"("Visible"=TRUE) -> ()  [unwired: 2 in, 2 out]
                n171 = property on="Test Slider" class="Slide (strict)"("Visible"=FALSE) -> ()  [unwired: 2 in, 2 out]
              }
              frame "Exposure Priority  **" {
                n172 = Index Array(array=w291, index=3) -> (element=w292:cluster{string[]})
                n173 = call <vilib>:"NT Read String.vi"("Name"=w294) -> ("String"=w293:string)  [unwired: 9 in, 1 out]
                n174 = Unbundle(w292) -> (w288:string[])
                n175 = Match First String(2:w288, 3:w293) -> (0:w289:i32)  [unwired: 1 out]
                n176 = property on="Test Ring" class="Ring (strict)"("Value"=w289, "Strings []"=w288) -> ()  [unwired: 2 in, 2 out]
                n177 = property on="Test Ring" class="Ring (strict)"("Visible"=TRUE) -> ()  [unwired: 2 in, 2 out]
                n178 = property on="Test Slider" class="Slide (strict)"("Visible"=FALSE) -> ()  [unwired: 2 in, 2 out]
              }
              frame "Color Enable  **" {
                n179 = Index Array(array=w300, index=4) -> (element=w301:cluster{string[]})
                n180 = call <vilib>:"NT Read String.vi"("Name"=w303) -> ("String"=w302:string)  [unwired: 9 in, 1 out]
                n181 = Unbundle(w301) -> (w297:string[])
                n182 = Match First String(2:w297, 3:w302) -> (0:w298:i32)  [unwired: 1 out]
                n183 = property on="Test Ring" class="Ring (strict)"("Value"=w298, "Strings []"=w297) -> ()  [unwired: 2 in, 2 out]
                n184 = property on="Test Ring" class="Ring (strict)"("Visible"=TRUE) -> ()  [unwired: 2 in, 2 out]
                n185 = property on="Test Slider" class="Slide (strict)"("Visible"=FALSE) -> ()  [unwired: 2 in, 2 out]
              }
              frame Default {
                n186 = property on="Test Ring" class="Ring (strict)"("Visible"=FALSE) -> ()  [unwired: 2 in, 2 out]
                n187 = property on="Test Slider" class="Slide (strict)"("Visible"=FALSE) -> ()  [unwired: 2 in, 2 out]
              }
              frame "Brightness  **", "Color Level  **", "Compression  **", "FPS  **", "Sharpness  **" {
                n188 = call <vilib>:"NT Read Number.vi"("Name"=w309) -> ("Numeric"=w308:dbl)  [unwired: 9 in, 1 out]
                n189 = local write "Test Slider"(w308) -> ()
                n190 = property on="Test Slider" class="Slide (strict)"("Visible"=TRUE, "Scale.Maximum"=100.0 ("Scale.Range:Maximum")) -> ()  [unwired: 2 in, 2 out]
                n191 = property on="Test Ring" class="Ring (strict)"("Visible"=FALSE) -> ()  [unwired: 2 in, 2 out]
              }
            }
          }
        }
        n192 = property on="Progress" class="Clust (strict)"("Visible"=FALSE) -> ()  [unwired: 2 in, 2 out]
      }
      event "Test Name": Mouse Enter {
        # "Populate the ring with the list of tests"
        n193 = event-data() -> ()  [unwired: 1 in, 1 out]
        n194 = call <vilib>:"NT Read String Array.vi"("Name"="/TestMode/TestList") -> ("String Array"=w318:string[])  [unwired: 9 in, 1 out]
        n195 = Build Array (concatenate)("Select the test to run...", w318) -> (w317:string[])
        n196 = property on="Test Name" class="Ring (strict)"("Strings []"=w317) -> ()  [unwired: 2 in, 2 out]
      }
      event "Test Name": Value Change {
        w321 = FALSE ("Visible")
        # "Tell the robot the test name to run"
        n197 = event-data() -> ("NewVal"=w325:u16)  [unwired: 1 in]
        n198 = property on="Test Name" class="Ring (strict)"() -> ("Strings []"=w326:string[])  [unwired: 2 in, 2 out]
        n199 = local write "Progress"(T7 {"Test Progress"=0, "Test Progress Text"=""} ("Progress")) -> ()
        n200 = Index Array(array=w326, index=w325) -> (element=w324:string)
        n201 = call <vilib>:"NT Write String.vi"("String"=w324, "Name"="/TestMode/TestName") -> ()  [unwired: 9 in, 1 out]
        n202 = property on="Progress" class="Clust (strict)"("Visible"=TRUE) -> ()  [unwired: 2 in, 2 out]
        n203 = property on="Motor" class="Clust (strict)"("Visible"=w321) -> ()  [unwired: 2 in, 2 out]
        n204 = property on="Test Slider" class="Slide (strict)"("Visible"=w321) -> ()  [unwired: 2 in, 2 out]
        n205 = property on="On/Off" class="Bool (strict)"("Visible"=w321) -> ()  [unwired: 2 in, 2 out]
        n206 = property on="Rev/Fwd" class="Clust (strict)"("Visible"=w321) -> ()  [unwired: 2 in, 2 out]
        n207 = property on="Test Ring" class="Ring (strict)"("Visible"=w321) -> ()  [unwired: 2 in, 2 out]
      }
      event "Select Auto": Mouse Enter {
        # "Populate the combo box with the list of autonomous options"
        n208 = event-data() -> ()  [unwired: 1 in, 1 out]
        n209 = call <vilib>:"NT Read String Array.vi"("Name"="Auto List") -> ("String Array"=w328:string[])  [unwired: 9 in, 1 out]
        n210 = property on="Select Auto" class="CmbBox"("Strings[]"=w328) -> ()  [unwired: 2 in, 2 out]
      }
      event "Select Auto": Value Change {
        # "User modified the Auto Selection. Write to NT variable so robot knows."
        n211 = event-data() -> ("NewVal"=w332:string)  [unwired: 1 in]
        n212 = call <vilib>:"NT Write String.vi"("String"=w332, "Name"="Auto Selector") -> ()  [unwired: 9 in, 1 out]
      }
      event "Command Selection": Value Change {
        # "Get the params and show in table"
        n213 = event-data() -> ("NewVal"=w339:i32)  [unwired: 1 in]
        n214 = property on="Command Selection" class="MCListbox (strict)"() -> ("ItemNames"=w337:string[][])  [unwired: 2 in, 2 out]
        n215 = call <vilib>:"WPI_DashboardUpdate Command Params.vi"("NewVal"=w339, "Commands"=w337, "Param Tbl"=w338) -> ()  [unwired: 8 in, 1 out]
      }
      event "Execute Command": Value Change {
        # "Started one, Unique ID holds\nresponse"
        n216 = event-data() -> ()  [unwired: 1 in, 1 out]
        n217 = property on="Command Selection" class="MCListbox (strict)"() -> ("ItemNames"=w351:string[][])  [unwired: 2 in, 2 out]
        n218 = Index Array(array=w351, index (row)="Command Selection", index (col)=0) -> (element=w349:string)
        n219 = call <vilib>:"Invoke Commands.vi"("Command Params"="Command Params", "Function Name"=w349) -> ("Params"=w345:u8, "Started"=w344:bool)  [unwired: 7 in, 1 out]
        n220 = Array Subset(array="Command Params", length (row)=w345) -> (w346:string[][])  [unwired: 3 in]
        n221 = Select(t="Executing" ("Cmd Status"), s=w344, f="" ("Cmd Status")) -> (s? t:f=→"Cmd Status":string)
      }
      event "Command Selection": Double Click {
        n222 = event-data() -> ("Row"=w361:i32)  [unwired: 1 in]
        n223 = property on="Command Selection" class="MCListbox (strict)"() -> ("ItemNames"=w364:string[][])  [unwired: 2 in, 2 out]
        n224 = local read "Command Params"() -> (w359:string[][])
        n225 = Index Array(array=w364, index (row)=w361, index (col)=0) -> (element=w362:string)
        n226 = call <vilib>:"Invoke Commands.vi"("Command Params"=w359, "Function Name"=w362) -> ("Params"=w358:u8, "Started"=w353:bool)  [unwired: 7 in, 1 out]
        n227 = Array Subset(array=w359, length (row)=w358) -> (w357:string[][])  [unwired: 3 in]
        n228 = Select(t="Executing" ("Cmd Status"), s=w353, f="" ("Cmd Status")) -> (s? t:f=w354:string)
        n229 = local write "Cmd Status"(w354) -> ()
      }
      event "CheckList": Double Click {
        # "Shift clears all"
        # "Update symbols on the listbox"
        n230 = event-data() -> ("PlatMods.Shift"=w367:bool, "Row"=w369:i32)  [unwired: 1 in]
        n231 = case shown="True" w367 {
          tunnel: w369 -> [w373 _]
          tunnel: 1 -> [w372 _]
          frame False {
            n232 = property on="CheckList" class="LstBox (strict)"() -> ("Item Symbols"=w371:i32[])  [unwired: 2 in, 2 out]
            n233 = Replace Array Subset(array=w371, new element=w372, index=w373) -> (w370:i32[])
            n234 = property on="CheckList" class="LstBox (strict)"("Item Symbols"=w370) -> ()  [unwired: 2 in, 2 out]
          }
          frame True {
            w374 = 0 ("Top Row")
            n235 = property on="CheckList" class="LstBox (strict)"() -> ("Number of Rows"=w376:u32)  [unwired: 2 in, 2 out]
            n236 = Initialize Array(0, w376) -> (w375:i32[])
            n237 = property on="CheckList" class="LstBox (strict)"("Top Row"=w374, "Value"=w374, "Item Symbols"=w375) -> ()  [unwired: 2 in, 2 out]
          }
        }
      }
      event "CheckList": Key Down {
        # "Update symbols on the listbox\nLeft and right keys check and uncheck"
        n238 = event-data() -> ("VKey"=w381:T22)  [unwired: 1 in]
        n239 = case shown="\"Left\", \"Right\"" w381 {
          selector: w381 -> [w386 _]
          tunnel: eventvkey."Left" ("VKey") -> [w384 _]
          frame "Left", "Right" {
            n240 = Equal?(x=w384, y=w386) -> (x = y?=w385:bool)
            n241 = Select(t=0, s=w385, f=1) -> (s? t:f=w387:i32)
            n242 = property on="CheckList" class="LstBox (strict)"() -> ("Item Symbols"=w390:i32[])  [unwired: 2 in, 2 out]
            n243 = Replace Array Subset(array=w390, new element=w387, index="CheckList") -> (w389:i32[])
            n244 = property on="CheckList" class="LstBox (strict)"("Item Symbols"=w389) -> ()  [unwired: 2 in, 2 out]
          }
          frame Default {
          }
        }
      }
      event "DB Camera Config": Value Change {
        # "Show or hide the cluster of controls, store in ini file"
        n245 = event-data() -> ("NewVal"=w395:bool)  [unwired: 1 in]
        n246 = case shown="False" w395 {
          tunnel: w394 -> [w404 _]
          tunnel: [w397 w415] -> w393
          tunnel: w392 -> [w396 w415]
          frame False {
            w411 = "Camera"
            w414 = FALSE ("Visible")
            n247 = local read "Camera Settings"() -> (w403:T2)
            n248 = Index Array(array=w404) -> (element=w407:cluster{string[]})  [unwired: 1 in]
            n249 = Unbundle(w403) -> ("Frame Rate"=w402:i32, "Compression"=w401:i32, "Size"=w405:u16)
            n250 = Unbundle(w407) -> (w406:string[])
            n251 = Index Array(array=w406, index=w405) -> (element=w400:string)
            n252 = call-poly <vilib>:"Write Key.vi"("section"=w411, "value"=w400, "key"="Size", "refnum"=w396) -> ("refnum out"=w413:T20)  [unwired: 2 in, 5 out]
            n253 = call-poly <vilib>:"Write Key.vi"("section"=w411, "value"=w402, "key"="FrameRate", "refnum"=w413) -> ("refnum out"=w412:T20)  [unwired: 1 in, 6 out]
            n254 = property on="Camera Settings" class="Clust (strict)"("Visible"=w414) -> ()  [unwired: 2 in, 2 out]
            n255 = local write "DB Camera Config"(w414) -> ()
            n256 = call-poly <vilib>:"Write Key.vi"("section"=w411, "value"=w401, "key"="Compression", "refnum"=w412) -> ("refnum out"=w398:T20)  [unwired: 1 in, 6 out]
            n257 = call <vilib>:"Close Config Data.vi"("refnum"=w398) -> ("file path"=w399:path)  [unwired: 2 in, 8 out]
            n258 = call <vilib>:"Open Config Data.vi"("configuration file path"=w399) -> ("refnum"=w397:T20)  [unwired: 8 in, 2 out]
          }
          frame True {
            n259 = property on="Camera Settings" class="Clust (strict)"("Visible"=TRUE) -> ()  [unwired: 2 in, 2 out]
          }
        }
      }
      event "Camera Settings": Value Change {
        # "Update summary string when any elements of DB camera change"
        n260 = event-data() -> ("NewVal"=w429:T2)  [unwired: 1 in]
        n261 = Index Array(array=w425) -> (element=w424:cluster{string[]})  [unwired: 1 in]
        n262 = Unbundle(w429) -> ("Frame Rate"=w420:i32, "Compression"=w419:i32, "Size"=w422:u16)
        n263 = Unbundle(w424) -> (w423:string[])
        n264 = Index Array(array=w423, index=w422) -> (element=w421:string)
        n265 = Format Into String(format string="%s   %dfps   %d%%", w421, w420, w419) -> (resulting string=w426:string)  [unwired: 2 in, 1 out]
        n266 = Build Array(w426) -> (w427:string[])
        n267 = property on="DB Camera Config" class="Bool (strict)"("Strings [4]"=w427) -> ()  [unwired: 2 in, 2 out]
      }
      event "Motor.Enable": Value Change {
        # "When the test mode otor enable helper is set, update that\ntree row item's value"
        n268 = event-data() -> ("NewVal"=w436:bool)  [unwired: 1 in]
        n269 = Unbundle("Motor") -> ("Value"=w435:dbl)  [unwired: 1 out]
        n270 = Select(t=w435, s=w436, f=0.0) -> (s? t:f=w433:dbl)
        n271 = call <vilib>:"NT Write Number.vi"("Numeric"=w433, "Name"=w432) -> ()  [unwired: 9 in, 1 out]
      }
      event "Test Slider": Value Change {
        # "When the test mode slider helper is set, update that\ntree row item's value"
        n272 = event-data() -> ("NewVal"=w440:dbl)  [unwired: 1 in]
        n273 = call <vilib>:"NT Write Number.vi"("Numeric"=w440, "Name"=w441) -> ()  [unwired: 9 in, 1 out]
      }
      event "On/Off": Value Change {
        # "When the test mode on/off helper value is set, update that\ntree row item's value"
        n274 = event-data() -> ("NewVal"=w446:bool)  [unwired: 1 in]
        n275 = Boolean To (0,1)(Boolean=w446) -> (0, 1=w445:i16)
        n276 = call <vilib>:"NT Write Number.vi"("Numeric"=w445, "Name"=w444) -> ()  [unwired: 9 in, 1 out]
      }
      event "Rev/Fwd": Value Change {
        # "When the test mode helper value for relays is set, update that\ntree row item's value"
        n277 = event-data() -> ("NewVal.Forward"=w455:bool, "NewVal.Reverse"=w454:bool)  [unwired: 1 in]
        n278 = Boolean To (0,1)(Boolean=w455) -> (0, 1=w451:i16)
        n279 = Boolean To (0,1)(Boolean=w454) -> (0, 1=w453:i16)
        n280 = Negate(x=w453) -> (-x=w452:i16)
        n281 = Add(x=w451, y=w452) -> (x+y=w450:i16)
        n282 = call <vilib>:"NT Write Number.vi"("Numeric"=w450, "Name"=w449) -> ()  [unwired: 9 in, 1 out]
      }
      event "Test Ring": Value Change {
        # "When a test mode helper value is selected from the ring,\nset the tree item's variable to the string value"
        n283 = event-data() -> ("NewVal"=w460:u16)  [unwired: 1 in]
        n284 = property on="Test Ring" class="Ring (strict)"() -> ("Strings []"=w461:string[])  [unwired: 2 in, 2 out]
        n285 = Index Array(array=w461, index=w460) -> (element=w459:string)
        n286 = call <vilib>:"NT Write String.vi"("String"=w459, "Name"=w458) -> ()  [unwired: 9 in, 1 out]
      }
      event "Rec Mode": Value Change {
        # "Update globals for recording mode and path to read log from.\nClear when logging and let NetworkTables set path for vision to\nuse."
        n287 = event-data() -> ("NewVal"=w473:enum32{"Stop", "Record", "Playback"})  [unwired: 1 in]
        n288 = global write "WPI_DashboardLogging Global.vi" "Logging Filename"(path "") -> ()
        n289 = global write "WPI_DashboardLogging Global.vi" "Recording"(w473) -> ()
        n290 = case shown="\"Playback\"" w473 {
          tunnel: w472 -> [_ w475 w484]
          tunnel: [_ _ w483] -> w469
          tunnel: [_ _ w482] -> _
          tunnel: w467 -> [_ _ w480]
          tunnel: cluster{i32, i32} {-250, 170} -> [_ _ w479]
          tunnel: [_ _ T23 {"Image Size"=TRUE, "Image Type"=TRUE, "Pixel Value"=TRUE, "ROI Information"=TRUE, "Zoom Factor"=FALSE} ("Image Information Shown:All Elements")] -> w465
          tunnel: [_ _ TRUE ("Zoom Factor")] -> w464
          tunnel: w463 -> [_ _ w476]
          frame Default {
          }
          frame "Stop", "Record" {
            # "Place Window too"
            n291 = invoke class="VI" method="FP.Close"(reference=w475) -> (reference out=w474:refnum<vi>)  [unwired: 2 in, 2 out]
            n292 = invoke class="VI" method="Abort VI"(reference=w474) -> ()  [unwired: 2 in, 3 out]
          }
          frame "Playback" {
            n293 = call "Open Playback Panel.vi"("Offset"=w479, "DB VI Ref"=w480, "Playback in"=w484) -> ("Playback out"=w481:refnum<vi>)  [unwired: 8 in]
            n294 = register-events(w481, w476) -> (reference out=w483:refnum<event-registration>, error out=w482:errorcluster)  [unwired: 2 in]
          }
        }
        n295 = property on="Camera Image" class="ImageControl"("Image Information Shown"=w465, "Image Information Visible"=w464) -> ()  [unwired: 2 in, 2 out]
        n296 = call <vilib>:"WPI_DashboardNT Log FieldName Cache.vi"("Operation"=enum16{"Lookup/Add", "Index", "Clear"}."Clear") -> ()  [unwired: 8 in, 3 out]
      }
      event Panel Close {
        w486 = enum32{"Stop", "Record", "Playback"}."Stop" ("Rec Mode")
        # "Playback window has been closed, abort"
        n297 = event-data() -> ()  [unwired: 1 in, 4 out]
        n298 = local write "Rec Mode"(w486) -> ()
        n299 = global write "WPI_DashboardLogging Global.vi" "Recording"(w486) -> ()
      }
      event Panel Close {
        # "Abort playback window and ourself"
        n300 = event-data() -> ()  [unwired: 1 in, 4 out]
        n301 = invoke class="VI" method="FP.Close"(reference=w492) -> (reference out=w491:refnum<vi>)  [unwired: 2 in, 2 out]
        n302 = invoke class="VI" method="Abort VI"(reference=w491) -> (error out=w490:errorcluster)  [unwired: 2 in, 2 out]
        n303 = invoke class="VI" method="Abort VI"(error in=w490) -> ()  [unwired: 2 in, 3 out]
      }
      event User Event {
        n304 = event-data() -> ("IDs"=w500:cluster{"RPC field ID":u16, "Unique ID":u16}, "String"=w499:string)  [unwired: 1 in]
        n305 = Bundle("IDs"=w500, "String"=w499) -> (w498:T9)  [unwired: 1 in]
        n306 = call <vilib>:"Retrieve RPC Response.vi"("RPC Response"=w498) -> ("Output"=w495:string[][])  [unwired: 10 in]
        n307 = Build Array (concatenate)(w493, w495) -> (w494:string[][])
        n308 = local write "Command Params"(w494) -> ()
        n309 = local write "Cmd Status"("" ("Cmd Status")) -> ()
      }
      event "Vision": Value Change {
        # "Enable/Disable Compression slider.\nHW USB is hard-coded into the camera"
        n310 = event-data() -> ("NewVal"=w507:u16)  [unwired: 1 in]
        n311 = Equal?(x=w507, y=u32 2 ("milliseconds to wait")) -> (x = y?=w505:bool)
        n312 = Select(t=T24."Disabled and Grayed Out" ("Disabled"), s=w505, f=T24."Enabled" ("Disabled")) -> (s? t:f=w502:T24)
        n313 = property on="Compression" class="Slide (strict)"("DisabledEnum"=w502) -> ()  [unwired: 2 in, 2 out]
      }
      event "Tree": Double Click {
        n314 = event-data() -> ("PlatMods"=w512:T27, "Tag"=w511:string)  [unwired: 1 in]
        n315 = Unbundle(w512) -> ("Shift"=w510:bool)  [unwired: 4 out]
        n316 = Not(x=w510) -> (.not. x?=w509:bool)
        n317 = call <vilib>:"NT Update Persistence.vi"("Persistence"=w509, "Name"=w511) -> ()  [unwired: 9 in, 1 out]
      }
    }
  }
  n318 = while {
    tunnel: w49 -> [w516]
    i -> [w519]
    stop <- FALSE stop-if-true
    n319 = Wait (ms)(milliseconds to wait=u32 100) -> ()  [unwired: 1 out]
    n320 = case shown="\"Playback\"" "Rec Mode" {
      tunnel: w519 -> [_ _ w534]
      tunnel: [u32 2829099 ("Base Color") u32 11141120 ("Target Color") w523] -> w515
      frame "Stop", Default {
        # "Reset the color, extra updates don't cost much"
      }
      frame "Record" {
      }
      frame "Playback" {
        # "Playback"
        n321 = Quotient & Remainder(x=w534, y=u32 50 ("milliseconds to wait")) -> (x-y*floor(x/y)=w530:u32)  [unwired: 1 out]
        n322 = Divide(x=w530, y=u32 50 ("milliseconds to wait")) -> (x/y=w527:dbl)
        n323 = Multiply(x=6.283185307179586, y=w527) -> (x*y=w532:dbl)
        n324 = Sine(x=w532) -> (sin(x)=w531:dbl)
        n325 = Absolute Value(x=w531) -> (abs(x)=w524:dbl)
        n326 = call "Interpolate RGB Color.vi"("Proportion"=w524, "Target Color"=u32 30976, "Base Color"=u32 2829099) -> ("Result Color"=w523:u32)  [unwired: 8 in]
      }
    }
    n327 = property class="Pane"(reference=w516, "PaneColor"=w515) -> ()  [unwired: 1 in, 2 out]
  }
  n328 = local write "Dashboard Tab"(T1."Drive" ("Dashboard Tab")) -> ()
  n329 = property on="On/Off" class="Bool (strict)"("Visible"=w17) -> ()  [unwired: 2 in, 2 out]
  n330 = property on="Motor" class="Clust (strict)"("Visible"=w17) -> ()  [unwired: 2 in, 2 out]
  n331 = property on="Progress" class="Clust (strict)"("Visible"=w17) -> ()  [unwired: 2 in, 2 out]
  n332 = property on="Test Ring" class="Ring (strict)"("Visible"=w17) -> ()  [unwired: 2 in, 2 out]
  n333 = property on="Rev/Fwd" class="Clust (strict)"("Visible"=w17) -> ()  [unwired: 2 in, 2 out]
  n334 = property on="Camera Settings" class="Clust (strict)"("Visible"=w17) -> ()  [unwired: 2 in, 2 out]
  n335 = local write "DB Camera Config"(w17) -> ()
  n336 = local write "Command Params"(string[][] [] ("Command Params")) -> ()
  n337 = global write "WPI_DashboardLogging Global.vi" "Recording"(w43) -> ()
  n338 = local write "Rec Mode"(w43) -> ()
  n339 = while "Key" {
    shift-right: [w536] -> _
    shift-left: string[][] [] ("Key") -> [w542]
    shift-right: [w540] -> _
    shift-left: string[][] [] ("Key") -> [w539]
    stop <- TRUE continue-if-true
    n340 = call-poly <vilib>:"NT Read Value.vi"("Name"="Key") -> ("String Array"=w543:string[])  [unwired: 9 in, 1 out]
    n341 = call-poly <vilib>:"NT Write Value.vi"("String"="File Name", "Name"="File Location") -> ()  [unwired: 9 in, 1 out]
    n342 = Array Size(array=w543) -> (size(s)=w545:i32)
    n343 = Divide(x=w545, y=2) -> (x/y=w544:dbl)
    n344 = for {
      N: w544 -> [_]
      tunnel: w543 -> [w565]
      tunnel: [w564] -> w537 mode=indexing
      i -> [w563]
      w562 = 2 ("length")
      n345 = Multiply(x=w562, y=w563) -> (x*y=w561:i32)
      n346 = Array Subset(array=w565, index=w561, length=w562) -> (w564:string[])
    }
    n347 = Equal?(x="Key", y=w542) -> (x = y?=w541:bool)
    n348 = case shown="False" w541 {
      tunnel: "Key" -> [w556 _]
      frame False {
        n349 = for {
          tunnel: w556 -> [w559] mode=indexing
          shift-right: [w558] -> w554
          shift-left: string[] [] ("String Array") -> [w560]
          n350 = Insert Into Array(array=w560, new element=w559) -> (w558:string[])  [unwired: 1 in]
        }
        n351 = call-poly <vilib>:"NT Write Value.vi"("String Array"=w554, "Name"="Key") -> ()  [unwired: 9 in, 1 out]
      }
      frame True {
      }
    }
    n352 = Not Equal?(x=w539, y=w537) -> (x != y?=w538:bool)
    n353 = case shown="False" w538 {
      tunnel: w539 -> [w552 _]
      tunnel: [w552 w553] -> w540
      tunnel: w537 -> [_ w553]
      tunnel: [w551 w553] -> w536
      tunnel: "Key" -> [w551 _]
      frame False {
      }
      frame True {
        n354 = local write "Key"(w553) -> ()
      }
    }
  }
  n355 = while {
    tunnel: u16 1741 ("timeout ms (25000)") -> [w567]
    stop <- FALSE stop-if-true
    n356 = TCP Create Listener(10:w567) -> (0:w566:errorcluster, 3:w568:refnum<k5>)  [unwired: 4 in, 1 out]
    n357 = case shown="No Error" w566 {
      selector: w566 -> [w570 _]
      tunnel: w568 -> [w571 _]
      frame No Error {
        n358 = while {
          tunnel: w571 -> [w574]
          tunnel: w570 -> [w573]
          stop <- FALSE stop-if-true
          n359 = TCP Wait On Listener(8:w573, 11:w574) -> (0:w575:errorcluster, 4:w576:refnum<k5>)  [unwired: 2 in, 3 out]
          n360 = local write "TCP"(w576) -> ()
          n361 = case shown="No Error" w575 {
            frame No Error {
            }
            frame Error {
              n362 = Wait (ms)(milliseconds to wait=u32 1000) -> ()  [unwired: 1 out]
            }
          }
        }
      }
      frame Error {
        n363 = Wait (ms)(milliseconds to wait=u32 1000) -> ()  [unwired: 1 out]
      }
    }
  }
  n364 = local write "Command Selection"(u16 0 ("milliseconds to wait")) -> ()
  n365 = while "Lights" {
    stop <- TRUE continue-if-true
    n366 = call-poly <vilib>:"NT Write Value.vi"("Boolean"="Test", "Name"="Response Test") -> ()  [unwired: 9 in, 1 out]
    n367 = call-poly <vilib>:"NT Read Value.vi"("Name"="LED Lights Connected") -> ("Boolean"=→"Lights Connected":bool)  [unwired: 9 in, 1 out]
  }
